vi "Debug Panel.vi"() -> ()   [LabVIEW 2011, in "Debug Variable Library.lvlib"]
uses:
  Debug Variable Library.lvlib
panel:
  out "Indicies":u32[](array[numeric])
  out "Data Array 2":dbl[](array[numeric])
  out "Bool Array 2":bool[](array[boolean])
  out "Number 1":dbl
  out "Number 3":dbl
  out "Number 2":dbl
  out "sec refs":dbl[](array[numeric])
  out "Bool Array":bool[](array[boolean])
  out "Channel Order":string[](array[string])
  out "Error Out":bool
  in  "stop":bool
  out "counts req":dbl[](array[numeric])
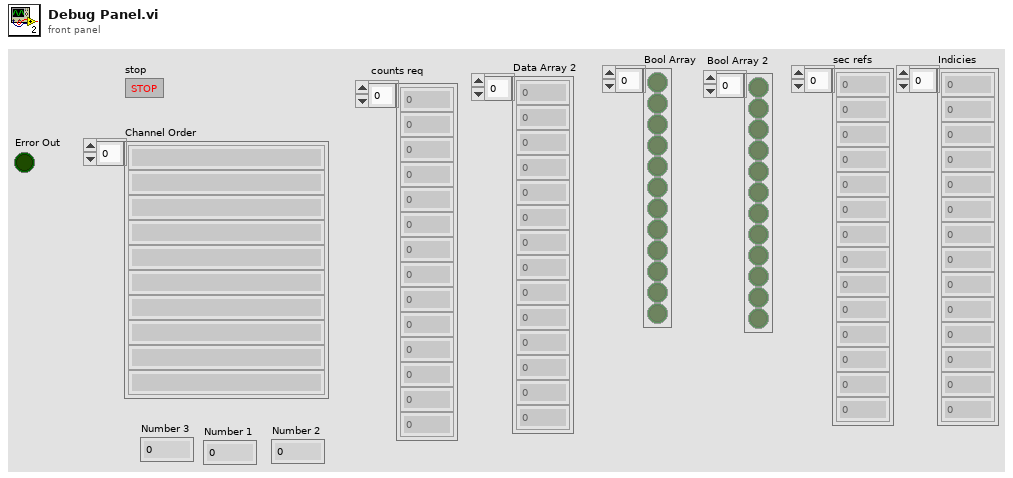
[diagram p1: front panel]
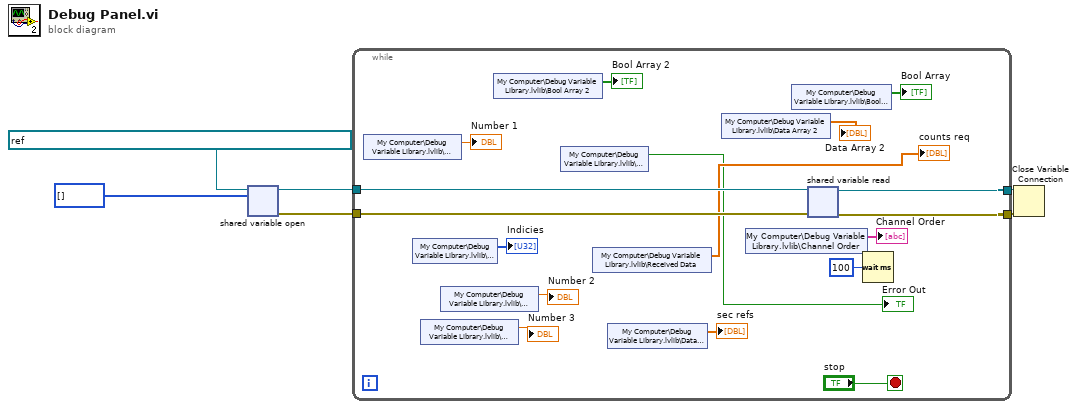
[diagram p0: block diagram]
diagram:
  n1 = shared-variable-open(refnum<k21> "ni.var.psp://localhost/Debug Variable Library/Received Data" ("shared variable refnum in"), u32[] []) -> (w3:refnum<k21>, w5:errorcluster)  [unwired: 2 in]
  n2 = while {
    tunnel: w5 -> [w23]
    tunnel: w3 -> [w22]
    tunnel: [w21] -> w2
    tunnel: [w20] -> w1
    stop <- "stop" stop-if-true
    n3 = shared-variable "My Computer\\Debug Variable Library.lvlib\\Number 1"() -> (→"Number 1":dbl)  [unwired: 1 in, 1 out]
    n4 = shared-variable "My Computer\\Debug Variable Library.lvlib\\Indicies"() -> (→"Indicies":u32[])  [unwired: 1 in, 1 out]
    n5 = shared-variable "My Computer\\Debug Variable Library.lvlib\\Number 3"() -> (→"Number 3":dbl)  [unwired: 1 in, 1 out]
    n6 = shared-variable "My Computer\\Debug Variable Library.lvlib\\Number 2"() -> (→"Number 2":dbl)  [unwired: 1 in, 1 out]
    n7 = shared-variable "My Computer\\Debug Variable Library.lvlib\\Bool Array 2"() -> (→"Bool Array 2":bool[])  [unwired: 1 in, 1 out]
    n8 = shared-variable "My Computer\\Debug Variable Library.lvlib\\Boolean"() -> (→"Error Out":bool)  [unwired: 1 in, 1 out]
    n9 = shared-variable "My Computer\\Debug Variable Library.lvlib\\Received Data"() -> (→"counts req":dbl[])  [unwired: 1 in, 1 out]
    n10 = shared-variable "My Computer\\Debug Variable Library.lvlib\\Data Array"() -> (→"sec refs":dbl[])  [unwired: 1 in, 1 out]
    n11 = shared-variable "My Computer\\Debug Variable Library.lvlib\\Data Array 2"() -> (→"Data Array 2":dbl[])  [unwired: 1 in, 1 out]
    n12 = shared-variable "My Computer\\Debug Variable Library.lvlib\\Channel Order"() -> (→"Channel Order":string[])  [unwired: 1 in, 1 out]
    n13 = shared-variable "My Computer\\Debug Variable Library.lvlib\\Bool Array"() -> (→"Bool Array":bool[])  [unwired: 1 in, 1 out]
    n14 = shared-variable-read(w22, w23) -> (w21:refnum<k21>, w20:errorcluster)  [unwired: 2 out]
    n15 = Wait (ms)(milliseconds to wait=u32 100) -> ()  [unwired: 1 out]
  }
  n16 = Close Variable Connection(8:w1, 11:w2) -> ()  [unwired: 1 out]
